vi "testSharedVariable.vi"() -> ()   [LabVIEW 2015]
uses:
  MasterStatus.ctl
  MySharedVariables.lvlib
panel:
  out "element":T1
  out "size(s)":i32
  in  "initit loop number":i32=5
  out "MasterStatusShared":T2
  in  "stop":bool
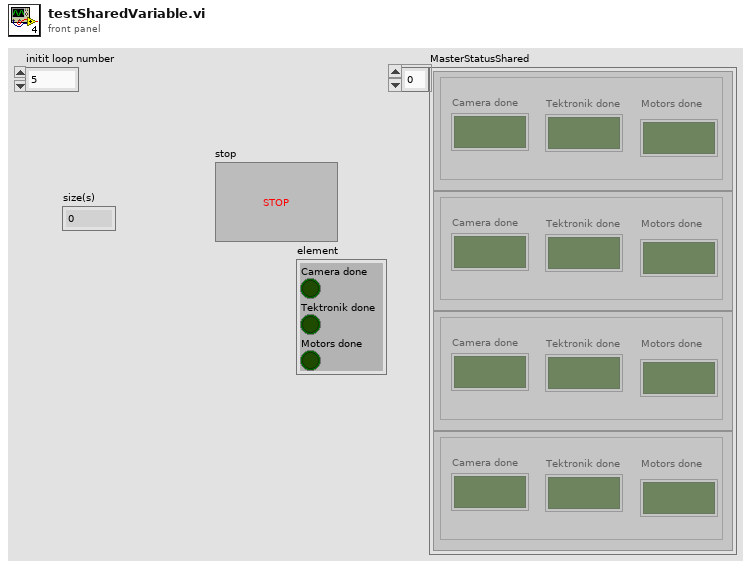
[diagram p1: front panel]
types:
  T1 = cluster{"Camera done":bool, "Tektronik done":bool, "Motors done":bool}
  T2 = typedef "MySharedVariables.lvlib/MasterStatus.ctl" = cluster{"Camera done":bool, "Tektronik done":bool, "Motors done":bool}[]
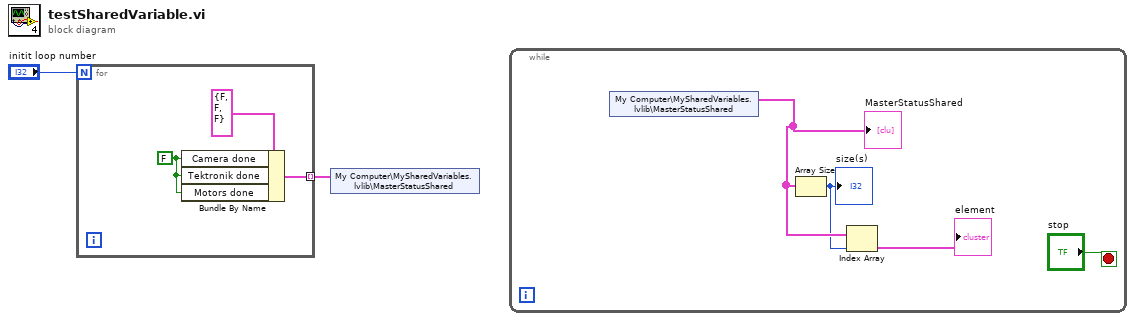
[diagram p0: block diagram]
diagram:
  n1 = for {
    N: "initit loop number" -> [_]
    tunnel: [w4] -> w1 mode=indexing
    w3 = FALSE ("Camera done")
    n2 = Bundle By Name(cluster=T1 {"Camera done"=FALSE, "Tektronik done"=FALSE, "Motors done"=FALSE} ("element"), "Camera done"=w3, "Tektronik done"=w3, "Motors done"=w3) -> (w4:T1)
  }
  n3 = shared-variable "My Computer\\MySharedVariables.lvlib\\MasterStatusShared"(w1) -> ()  [unwired: 1 in, 1 out]
  n4 = while {
    stop <- "stop" stop-if-true
    n5 = shared-variable "My Computer\\MySharedVariables.lvlib\\MasterStatusShared"() -> (w8:T2)  [unwired: 1 in, 1 out]
    "MasterStatusShared" <- w8
    n6 = Array Size(array=w8) -> (size(s)=w7:i32)
    "size(s)" <- w7
    n7 = Index Array(array=w8, index=w7) -> (element=→"element":T1)
  }
